vi "Init Server.vi"(6 "Descriptions":string[][](array[string]), 7 "trust all clients":bool=TRUE, 8 "error in (no error)":errorcluster, 9 "Parameters":T1[](array[typedef]) {"data type" items=["Boolean"=1, "SByte"=2, "Byte"=3, "Int16"=4, "UInt16"=5, "Int32"=6, "UInt32"=7, "Int64"=8, "UInt64"=9, "Float"=10, "Double"=11, "String"=12, "DateTime"=13, "ByteString"=15, "Array of Boolean"=101, "Array of SByte"=102, "Array of Byte"=103, "Array of Int16"=104, "Array of UInt16"=105, "Array of Int32"=106, "Array of UInt32"=107, "Array of Int64"=108, "Array of UInt64"=109, "Array of Float"=110, "Array of Double"=111, "Array of String"=112, "Array of DateTime"=113, "Array of ByteString"=115, "Matrix of Boolean"=201, "Matrix of SByte"=202, "Matrix of Byte"=203, "Matrix of Int16"=204, "Matrix of UInt16"=205, "Matrix of Int32"=206, "Matrix of UInt32"=207, "Matrix of Int64"=208, "Matrix of UInt64"=209, "Matrix of Float"=210, "Matrix of Double"=211, "Matrix of String "=212, "Matrix of DateTime"=213, "Matrix of ByteString"=215]}, 10 "supported security policies (None)":T8={"None"=TRUE, "Sign with Basic128Rsa15"=TRUE, "Sign and Encrypt with Basic128Rsa15"=TRUE, "Sign with Basic256"=TRUE, "Sign and Encrypt with Basic256"=TRUE}, 11 "OPC UA":T5 {"OPC tags"."data type" items=["Boolean"=1, "SByte"=2, "Byte"=3, "Int16"=4, "UInt16"=5, "Int32"=6, "UInt32"=7, "Int64"=8, "UInt64"=9, "Float"=10, "Double"=11, "String"=12, "DateTime"=13, "ByteString"=15, "Array of Boolean"=101, "Array of SByte"=102, "Array of Byte"=103, "Array of Int16"=104, "Array of UInt16"=105, "Array of Int32"=106, "Array of UInt32"=107, "Array of Int64"=108, "Array of UInt64"=109, "Array of Float"=110, "Array of Double"=111, "Array of String"=112, "Array of DateTime"=113, "Array of ByteString"=115, "Matrix of Boolean"=201, "Matrix of SByte"=202, "Matrix of Byte"=203, "Matrix of Int16"=204, "Matrix of UInt16"=205, "Matrix of Int32"=206, "Matrix of UInt32"=207, "Matrix of Int64"=208, "Matrix of UInt64"=209, "Matrix of Float"=210, "Matrix of Double"=211, "Matrix of String "=212, "Matrix of DateTime"=213, "Matrix of ByteString"=215]}) -> (0 "error out":errorcluster, 2 "server endpoint URL":string, 3 "OPC UA out":T5 {"OPC tags"."data type" items=["Boolean"=1, "SByte"=2, "Byte"=3, "Int16"=4, "UInt16"=5, "Int32"=6, "UInt32"=7, "Int64"=8, "UInt64"=9, "Float"=10, "Double"=11, "String"=12, "DateTime"=13, "ByteString"=15, "Array of Boolean"=101, "Array of SByte"=102, "Array of Byte"=103, "Array of Int16"=104, "Array of UInt16"=105, "Array of Int32"=106, "Array of UInt32"=107, "Array of Int64"=108, "Array of UInt64"=109, "Array of Float"=110, "Array of Double"=111, "Array of String"=112, "Array of DateTime"=113, "Array of ByteString"=115, "Matrix of Boolean"=201, "Matrix of SByte"=202, "Matrix of Byte"=203, "Matrix of Int16"=204, "Matrix of UInt16"=205, "Matrix of Int32"=206, "Matrix of UInt32"=207, "Matrix of Int64"=208, "Matrix of UInt64"=209, "Matrix of Float"=210, "Matrix of Double"=211, "Matrix of String "=212, "Matrix of DateTime"=213, "Matrix of ByteString"=215]})   [LabVIEW 2019, in "OPC addons.lvlib"]
uses:
  OPC addons.lvlib
  <vilib>/OPCUA/controls/Supported Security Policies.ctl
  OPC UA Server.ctl
  <vilib>/OPCUA/controls/OPC UA Server Refnum.ctl
  <vilib>/OPCUA/controls/NodeId.ctl
  OPC tag.ctl
  <vilib>/OPCUA/controls/Data Type.ctl
  Access level.ctl
  Period.ctl
  <vilib>/OPCUA/controls/Condition Type.ctl
  <vilib>/OPCUA/controls/Write Status.ctl
  <vilib>/OPCUA/server/Write Byte String Array.vi
  <vilib>/OPCUA/NI OPC UA Server.lvlib
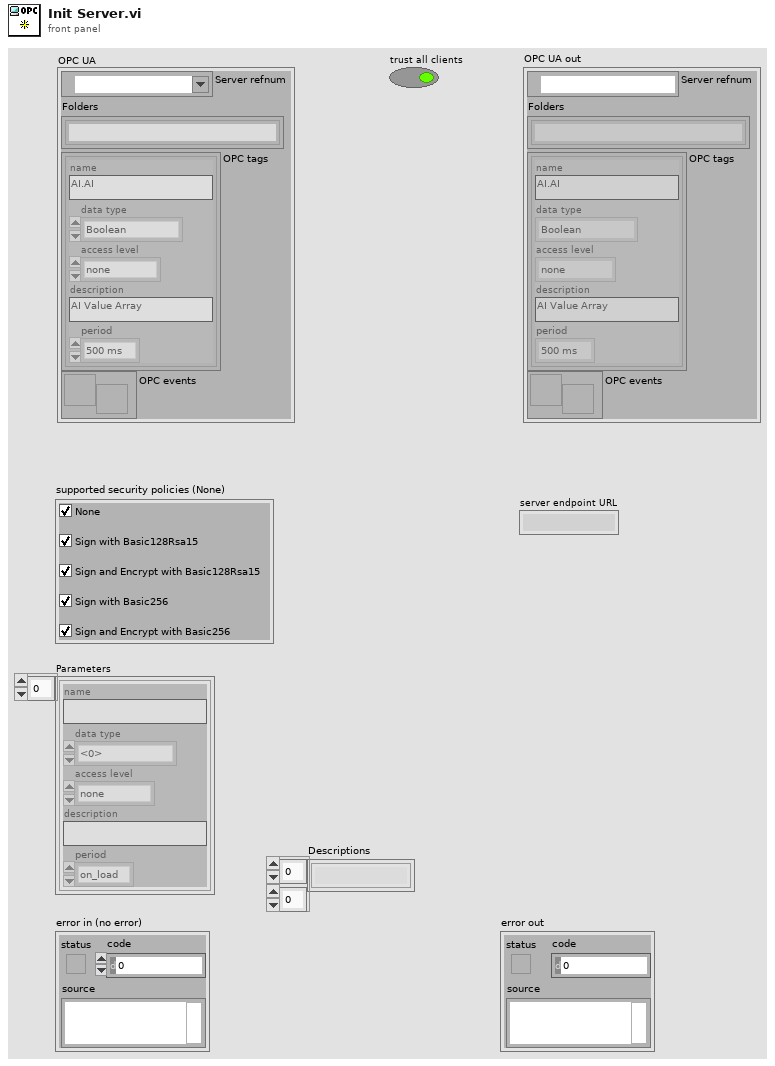
[diagram p1: front panel]
types:
  T1 = typedef "OPC addons.lvlib/OPC tag.ctl" = cluster{"name":string, "data type":T2, "access level":T3, "description":string, "period":T4}
  T2 = typedef "Data Type.ctl" = u16
  T3 = typedef "OPC addons.lvlib/Access level.ctl" = enum16{"none", "read-only", "write-only", "read/write"}
  T4 = typedef "OPC addons.lvlib/Period.ctl" = enum16{"on_load", "100 ms", "500 ms", "1 s"}
  T5 = typedef "OPC addons.lvlib/OPC UA Server.ctl" = cluster{"Server refnum":T6, "Folders":T7[], "OPC tags":T1[], "OPC events":refnum<user-event>}
  T6 = typedef "OPC UA Server Refnum.ctl" = refnum<k21>
  T7 = typedef "NodeId.ctl" = string
  T8 = typedef "Supported Security Policies.ctl" = cluster{"None":bool, "Sign with Basic128Rsa15":bool, "Sign and Encrypt with Basic128Rsa15":bool, "Sign with Basic256":bool, "Sign and Encrypt with Basic256":bool}
  T9 = typedef "Write Status.ctl" = u32
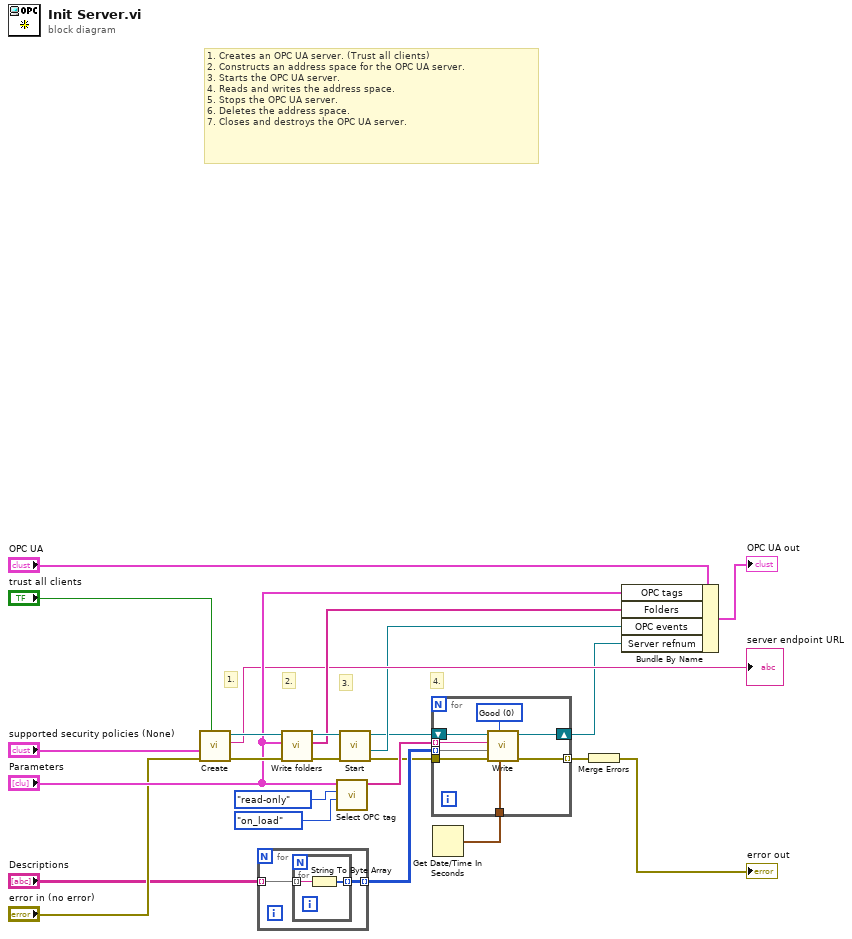
[diagram p0: block diagram]
diagram:
  # "2."
  # "3."
  # "1."
  # "4."
  # "1. Creates an OPC UA server. (Trust all clients)\n2. Constructs an address space for the OPC UA server.\n3. Starts the OPC UA server.\n4. Reads and writes the address space.\n5. Stops the OPC UA server.\n6. Deletes the address space.\n7. Closes and destroys the OPC UA server."
  n1 = call <vilib>:"Create.vi"("trust all clients (F)"="trust all clients", "error in (no error)"="error in (no error)", "supported security policies (None)"="supported security policies (None)") -> ("error out"=w21:errorcluster, "server endpoint URL"=→"server endpoint URL":string, "OPC UA server refnum out"=w22:T6)  [unwired: 6 in]
  n2 = for {
    tunnel: "Descriptions" -> [w26] mode=indexing
    tunnel: [w25] -> w6 mode=indexing
    n3 = for {
      tunnel: w26 -> [w28] mode=indexing
      tunnel: [w27] -> w25 mode=indexing
      n4 = String To Byte Array(string=w28) -> (unsigned byte array=w27:u8[])
    }
  }
  n5 = call "Write folders.vi"("error in (no error)"=w21, "Parameters"="Parameters", "OPC UA server refnum in"=w22) -> ("error out"=w19:errorcluster, "Folders"=w15:T7[], "OPC UA server refnum out"=w20:T6)  [unwired: 6 in]
  n6 = call "Select OPC tag.vi"("period"=Period."on_load", "access level"=Access_level."read-only", "OPC Params"="Parameters") -> ("tags"=w18:string[])  [unwired: 8 in]
  n7 = call <vilib>:"Start.vi"("error in (no error)"=w19, "OPC UA server refnum in"=w20) -> ("error out"=w1:errorcluster, "condition response event refnum"=w3:refnum<user-event>, "OPC UA server refnum out"=w2:T6)  [unwired: 7 in]
  n8 = Get Date/Time In Seconds() -> (seconds since 1Jan1904=w24:timestamp)
  n9 = for {
    tunnel: w6 -> [w29] mode=indexing
    tunnel: w24 -> [w31]
    tunnel: w1 -> [w34]
    tunnel: [w33] -> w23 mode=indexing
    tunnel: w18 -> [w30] mode=indexing
    shift-right: [w35] -> w4
    shift-left: w2 -> [w36]
    w32 = T9 0 items=["Good"=0, "Uncertain"=1073741824, "Uncertain_InitialValue"=1083310080, "Uncertain_LastUsableValue"=1083179008, "Uncertain_SensorNotAccurate"=1083375616, "Uncertain_EngineeringUnitsExceeded"=1083441152, "Bad"=2147483648, "Bad_NoCommunication"=2150694912, "Bad_NotReadable"=2151284736, "Bad_NotWritable"=2151350272, "Bad_OutOfRange"=2151415808, "Bad_WaitingForInitialData"=2150760448] ("node status")
    n10 = call-poly <vilib>:"Write.vi"("timestamp (current time)"=w31, "node status"=w32, "error in (no error)"=w34, "values"=w29, "node ID"=w30, "OPC UA server refnum in"=w36) -> ("error out"=w33:errorcluster, "OPC UA server refnum out"=w35:T6)  [unwired: 3 in, 1 out]
  }
  n11 = Merge Errors(w23) -> (→"error out":errorcluster)
  n12 = Bundle By Name(cluster="OPC UA", "OPC tags"="Parameters", "Folders"=w15, "OPC events"=w3, "Server refnum"=w4) -> (→"OPC UA out":T5)
